vi "Convert Data Bytes to Calibration number.vi"(11 "Data Bytes":u8[](array[numeric])) -> (3 "Calibration Release Number":string)   [LabVIEW 2025]
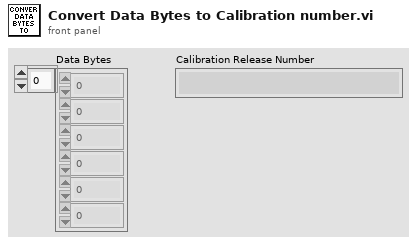
[diagram p1: front panel]
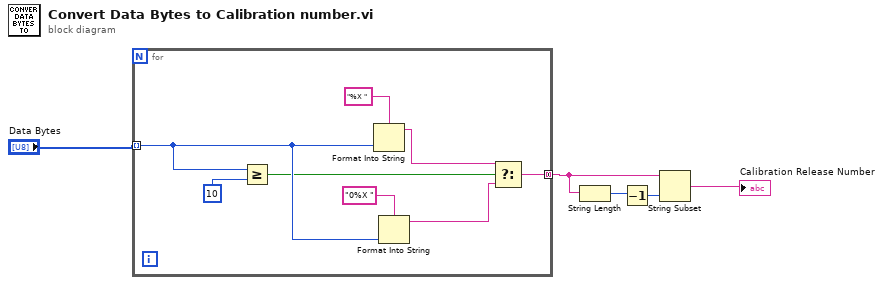
[diagram p0: block diagram]
diagram:
  n1 = for {
    tunnel: "Data Bytes" -> [w11] mode=indexing
    tunnel: [w8] -> w3 mode=concatenating
    n2 = Greater Or Equal?(x=w11, y=u8 10) -> (x >= y?=w10:bool)
    n3 = Format Into String(format string="%X ", w11) -> (resulting string=w9:string)  [unwired: 2 in, 1 out]
    n4 = Format Into String(format string="0%X ", w11) -> (resulting string=w6:string)  [unwired: 2 in, 1 out]
    n5 = Select(t=w9, s=w10, f=w6) -> (s? t:f=w8:string)
  }
  n6 = String Length(string=w3) -> (length=w2:i32)
  n7 = Decrement(x=w2) -> (x-1=w1:i32)
  n8 = String Subset(string=w3, length (rest)=w1) -> (substring=→"Calibration Release Number":string)  [unwired: 1 in]
